vi "Wait for Time.vi"(0 "future time (ns)":u64) -> (1 "time snapped event":bool, 2 "time already elapsed":bool, 3 "return time (ns)":u64)   [LabVIEW 2013, in "FPGA Timekeeper.lvlib"]
doc: "Waits for the given time to arrive."
uses:
  FPGA Timekeeper.lvlib
  <vilib>/Platform/TimedLoop/XDataNode/timing_clust.ctl
  <vilib>/Platform/TimedLoop/XDataNode/nitl_modes.ctl
  <vilib>/Platform/TimedLoop/XDataNode/wakeup.ctl
  private/time adjustment event (g).vi
  <vilib>/rvi/Emulation/niFpgaSctlEmulationGetInTimedLoop.vi
  <vilib>/rvi/Emulation/niFpgaEmulationReportErrorSimple.vi
  <vilib>/rvi/Emulation/niFpgaGetClockAttributes.vi
  <vilib>/rvi/Emulation/niFpgaCriticalErrorInLSC.vi
  <vilib>/Platform/TimedLoop/XDataNode/XDataNode.xnode
  <vilib>/Platform/TimedLoop/XDataNode/XDNodeRunTimeDep.lvlib
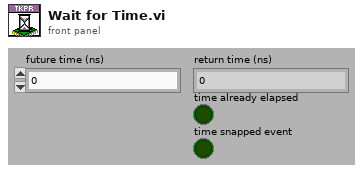
[diagram p1: front panel]
types:
  T1 = typedef "XDNodeRunTimeDep.lvlib/timing_clust.ctl" = cluster{"Expected End [f-1]":u64, "Actual End [f-1]":u64, "Finished Late? [f-1]":bool, "Expected End [i-1]":u64, "Actual End [i-1]":u64, "Finished Late? [i-1]":bool, "Expected Start [i]":u64, "Actual Start [i]":u64, "Expected Start [f]":u64, "Actual Start [f]":u64, "Source Name":string, "Structure Name":string, "Period":i64, "Deadline":i64, "Offset":i64, "Start":i64, "Priority":i32, "Timeout":i32, "Mode":T2, "Wakeup Reason":T3, "Error":errorcluster, "Source Type":string, "Secondary Source Type":string, "Global End Time":u64, "Global Start Time":u64, "Frame Duration":u64, "Iteration Duration":u64, "Assigned CPU":i32, "I/O Scan Engine Mode":u32}
  T2 = typedef "XDNodeRunTimeDep.lvlib/nitl_modes.ctl" = enum32{"No Change", "Process missed periods, maintain original phase", "Discard missed periods, maintain original phase", "Process missed periods, ignore original phase", "Discard missed periods, ignore original phase"}
  T3 = typedef "XDNodeRunTimeDep.lvlib/wakeup.ctl" = enum32{"Normal", "Aborted", "Asynchronous wakeup", "Timing source error", "Timed loop error", "Timeout"}
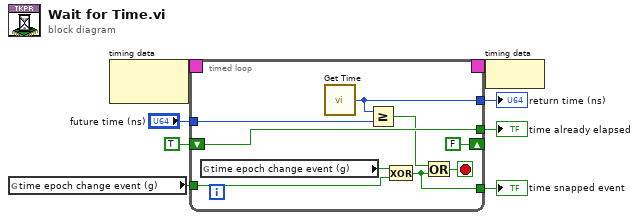
[diagram p0: block diagram]
diagram:
  n1 = global read "time adjustment event (g).vi" "time epoch change event (g)"() -> (w2:bool)
  n2 = node-c288() -> (w8:T1)  [unwired: 1 in]
  n3 = timed-loop {
    timing: w8 -> [_]
    timing-out: [_] -> w7
    shift-right: [FALSE] -> _
    shift-left: TRUE -> [w17]
    tunnel: [w17] -> w6
    tunnel: "future time (ns)" -> [w16]
    tunnel: [w15] -> w4
    tunnel: w2 -> [w13]
    tunnel: [w11] -> w1
    stop <- w12 stop-if-true
    n4 = global read "time adjustment event (g).vi" "time epoch change event (g)"() -> (w14:bool)
    n5 = call "Get Time.vi"() -> ("time (ns)"=w15:u64)
    n6 = Greater Or Equal?(x=w15, y=w16) -> (x >= y?=w10:bool)
    n7 = Exclusive Or(1:w13, 2:w14) -> (0:w11:bool)
    n8 = Or(x=w10, y=w11) -> (x .or. y?=w12:bool)
  }
  "time already elapsed" <- w6
  "return time (ns)" <- w4
  "time snapped event" <- w1
  n9 = node-c288(w7) -> ()
